vi "Gateway_SetThisHostAddr.vi"(0 "GatewayClass in":refnum<class "GatewayClass.lvclass">, 5 "This Hostname":string, 7 "MIDAS Address":string, 9 "MIDAS Port Number":u16, 11 "error in (no error)":errorcluster) -> (4 "GatewayClass out":refnum<class "GatewayClass.lvclass">, 15 "error out":errorcluster)   [LabVIEW 2018, in "GatewayClass.lvclass"]
uses:
  GatewayClass.lvclass
  GatewayClass.lvclass/GatewayClass.ctl
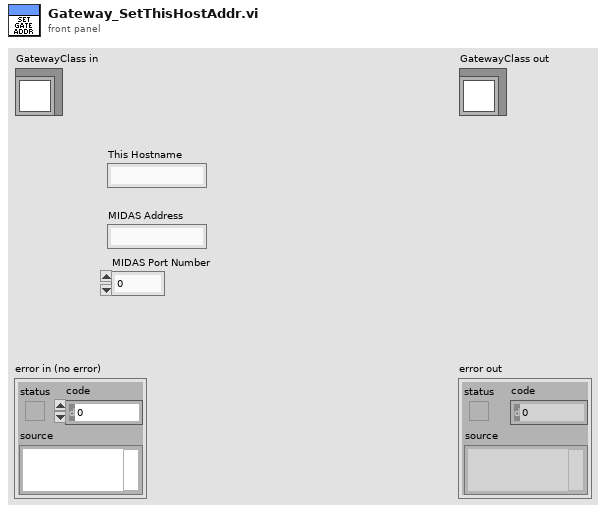
[diagram p1: front panel]
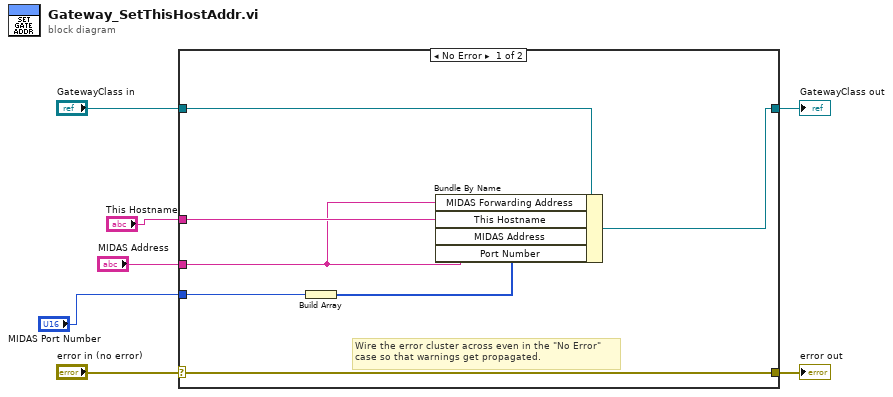
[diagram p0: block diagram]
diagram:
  n1 = case shown="No Error" "error in (no error)" {
    selector: "error in (no error)" -> [w14 w16]
    tunnel: [w14 w16] -> w6
    tunnel: [w12 w15] -> w4
    tunnel: "GatewayClass in" -> [w13 w15]
    tunnel: "This Hostname" -> [w11 _]
    tunnel: "MIDAS Address" -> [w8 _]
    tunnel: "MIDAS Port Number" -> [w9 _]
    frame No Error {
      # "Wire the error cluster across even in the \"No Error\"\ncase so that warnings get propagated."
      n2 = Build Array(w9) -> (w10:u16[])
      n3 = Bundle By Name(cluster=w13, "MIDAS Forwarding Address"=w8, "This Hostname"=w11, "MIDAS Address"=w8, "Port Number"=w10) -> (w12:refnum<class "GatewayClass.lvclass">)
    }
    frame Error {
    }
  }
  "error out" <- w6
  "GatewayClass out" <- w4
